vi "UnlockProtectiveStop.vi"(0 "Universal Robot.lvclass in":refnum<class "Universal Robot.lvclass">, 5 "error in (no error)":errorcluster) -> (14 "Universal Robot.lvclass out":refnum<class "Universal Robot.lvclass">, 19 "error out":errorcluster)   [LabVIEW 2019, in "Universal Robot.lvclass"]
uses:
  Universal Robot.lvclass
  Universal Robot.lvclass/Universal Robot.ctl
  Client Interfaces/Dashboard Server/Dashboard Server.lvclass
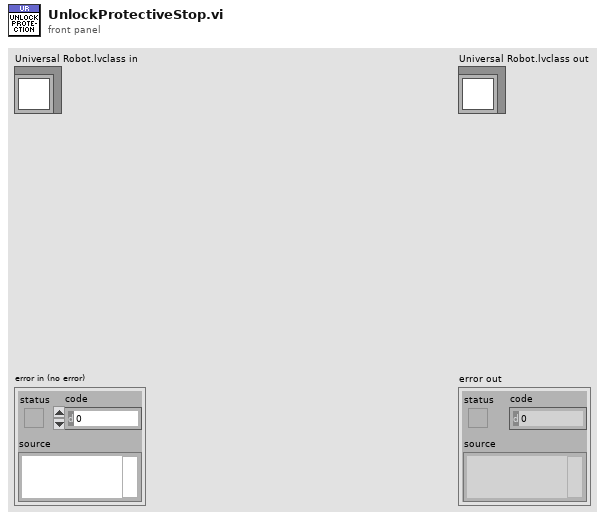
[diagram p1: front panel]
types:
  T1 = typedef "Universal Robot.lvclass/SafetyStatus.ctl" = enum16{"INVALID", "NORMAL", "REDUCED", "PROTECTIVE_STOP", "RECOVERY", "SAFEGUARD_STOP", "SYSTEM_EMERGENCY_STOP", "ROBOT_EMERGENCY_STOP", "VIOLATION", "FAULT", "AUTOMATIC_MODE_SAFEGAURD_STOP", "SYSTEM_THREE_POSITION_ENABLING_STOP"}
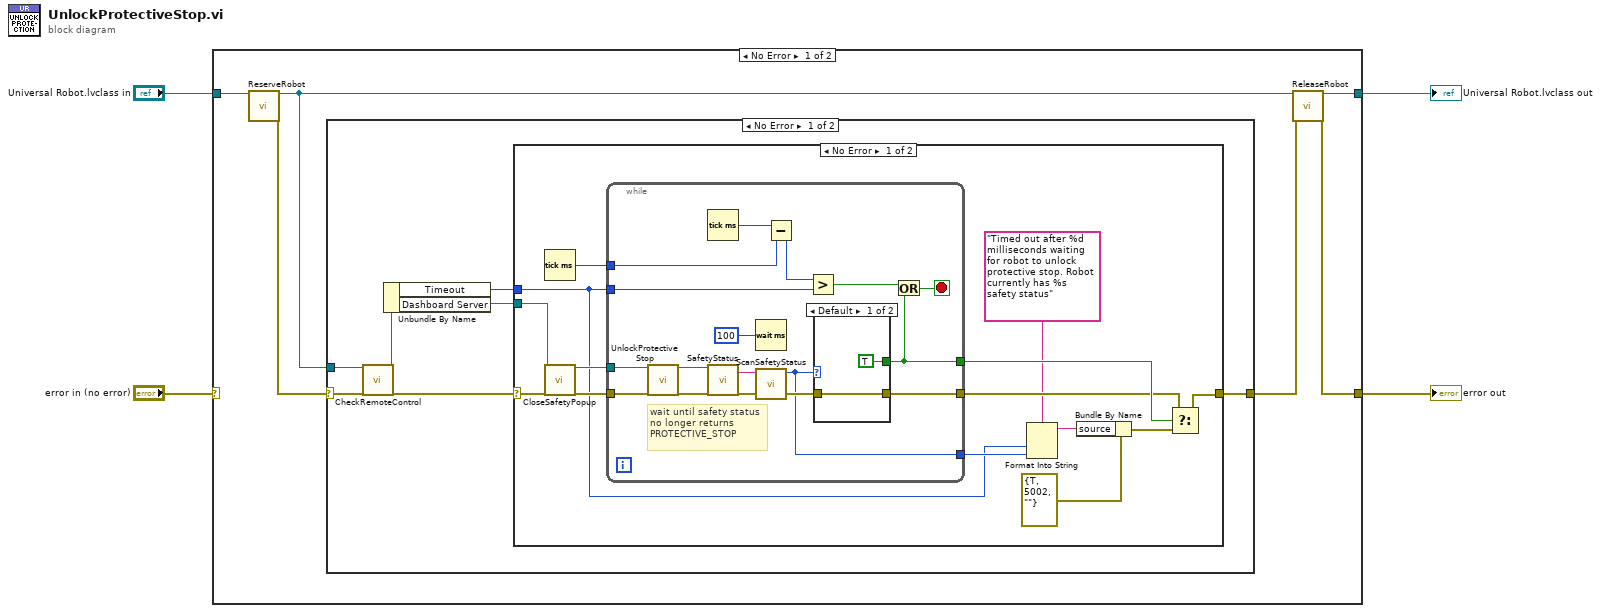
[diagram p0: block diagram]
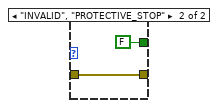
[diagram p2: hidden frame]
diagram:
  n1 = case shown="No Error" "error in (no error)" {
    selector: "error in (no error)" -> [_ w55]
    tunnel: [w6 w55] -> w3
    tunnel: "Universal Robot.lvclass in" -> [w10 w54]
    tunnel: [w8 w54] -> w1
    frame No Error {
      n2 = call "ReserveRobot.vi"("Universal Robot.lvclass in"=w10) -> ("Universal Robot.lvclass out"=w9:refnum<class "Universal Robot.lvclass">, "error out"=w5:errorcluster)  [unwired: 17 in]
      n3 = case shown="No Error" w5 {
        selector: w5 -> [w11 w53]
        tunnel: w9 -> [w13 _]
        tunnel: [w12 w53] -> w7
        frame No Error {
          n4 = call-dynamic "CheckRemoteControl.vi"("Universal Robot.lvclass in"=w13, "error in (no error)"=w11) -> ("Universal Robot.lvclass out"=w17:refnum<class "Universal Robot.lvclass">, "error out"=w14:errorcluster)  [unwired: 16 in]
          n5 = Unbundle By Name(w17) -> ("Timeout"=w15:u32, "Dashboard Server"=w16:refnum<class "Dashboard Server.lvclass">)
          n6 = case shown="No Error" w14 {
            selector: w14 -> [w22 w52]
            tunnel: [w31 w52] -> w12
            tunnel: w16 -> [w21 _]
            tunnel: w15 -> [w18 _]
            frame No Error {
              n7 = Tick Count (ms)() -> (millisecond timer value=w30:u32)
              n8 = call-dynamic "CloseSafetyPopup.vi"("DashboardServer in"=w21, "error in (no error)"=w22) -> ("DashboardServer out"=w20:refnum<class "Dashboard Server.lvclass">, "error out"=w19:errorcluster)  [unwired: 15 in, 1 out]
              n9 = while {
                tunnel: w18 -> [w47]
                tunnel: w30 -> [w46]
                tunnel: [w33] -> w29
                tunnel: [w32] -> w27
                tunnel: w20 -> [w45]
                tunnel: w19 -> [w44]
                tunnel: [w34] -> w28
                stop <- w36 stop-if-true
                # "wait until safety status no longer returns PROTECTIVE_STOP"
                n10 = call-dynamic "UnlockProtectiveStop.vi"("DashboardServer in"=w45, "error in (no error)"=w44) -> ("DashboardServer out"=w42:refnum<class "Dashboard Server.lvclass">, "error out"=w43:errorcluster)  [unwired: 15 in, 1 out]
                n11 = Tick Count (ms)() -> (millisecond timer value=w40:u32)
                n12 = call-dynamic "SafetyStatus.vi"("DashboardServer in"=w42, "error in (no error)"=w43) -> ("safetyStatus"=w37:string, "error out"=w35:errorcluster)  [unwired: 15 in, 1 out]
                n13 = Wait (ms)(milliseconds to wait=u32 100) -> ()  [unwired: 1 out]
                n14 = call "ScanSafetyStatus.vi"("safetyStatus in"=w37) -> ("safetyStatus out"=w32:T1)  [unwired: 10 in]
                n15 = Subtract(x=w40, y=w46) -> (x-y=w39:u32)
                n16 = Greater?(x=w39, y=w47) -> (0:w38:bool)
                n17 = case shown="Default" w32 {
                  tunnel: w35 -> [w49 w51]
                  tunnel: [w49 w51] -> w34
                  tunnel: [TRUE FALSE] -> w33
                  frame Default {
                  }
                  frame "INVALID", "PROTECTIVE_STOP" {
                  }
                }
                n18 = Or(x=w38, y=w33) -> (x .or. y?=w36:bool)
              }
              n19 = Format Into String(format string="Timed out after %d milliseconds waiting for robot to unlock protective stop. Robot currently has %s safety status", w18, w27) -> (resulting string=w25:string)  [unwired: 2 in, 1 out]
              n20 = Bundle By Name(cluster=errorcluster {"status"=TRUE, "code"=5002, "source"=""} ("error constant"), "source"=w25) -> (w24:errorcluster)
              n21 = Select(t=w28, s=w29, f=w24) -> (s? t:f=w31:errorcluster)
            }
            frame Error {
            }
          }
        }
        frame Error {
        }
      }
      n22 = call "ReleaseRobot.vi"("Universal Robot.lvclass in"=w9, "error in (no error)"=w7) -> ("Universal Robot.lvclass out"=w8:refnum<class "Universal Robot.lvclass">, "error out"=w6:errorcluster)  [unwired: 16 in]
    }
    frame Error {
    }
  }
  "error out" <- w3
  "Universal Robot.lvclass out" <- w1
